vi "Draw Shapes.vi"(0 "Picture in":refnum<vi>, 1 "Commands":cluster{"Time (s)":dbl, T2, "Enabled":bool}[](array[cluster]), 3 "Sample Period (s)":dbl=0.02, 5 "Points":cluster{"x":dbl, "y":dbl, "th":dbl}[](array[cluster]), 6 "Path Points MEGA":cluster{"x":dbl, "y":dbl}[][](array[cluster]), 9 "new picture in":picture, 10 "Output Point MEGA":T1(array[cluster]), 11 "Results":T5, 12 "Output Point":T4, 14 "Path Points":cluster{"x":dbl, "y":dbl}[](array[cluster]), 15 "MEGA?":bool) -> (4 "new picture out":picture)   [LabVIEW 2025]
uses:
  Types/Single Cmd Info.ctl
  <vilib>/picture/picture.llb/imagedata.ctl
  Global Settings.vi
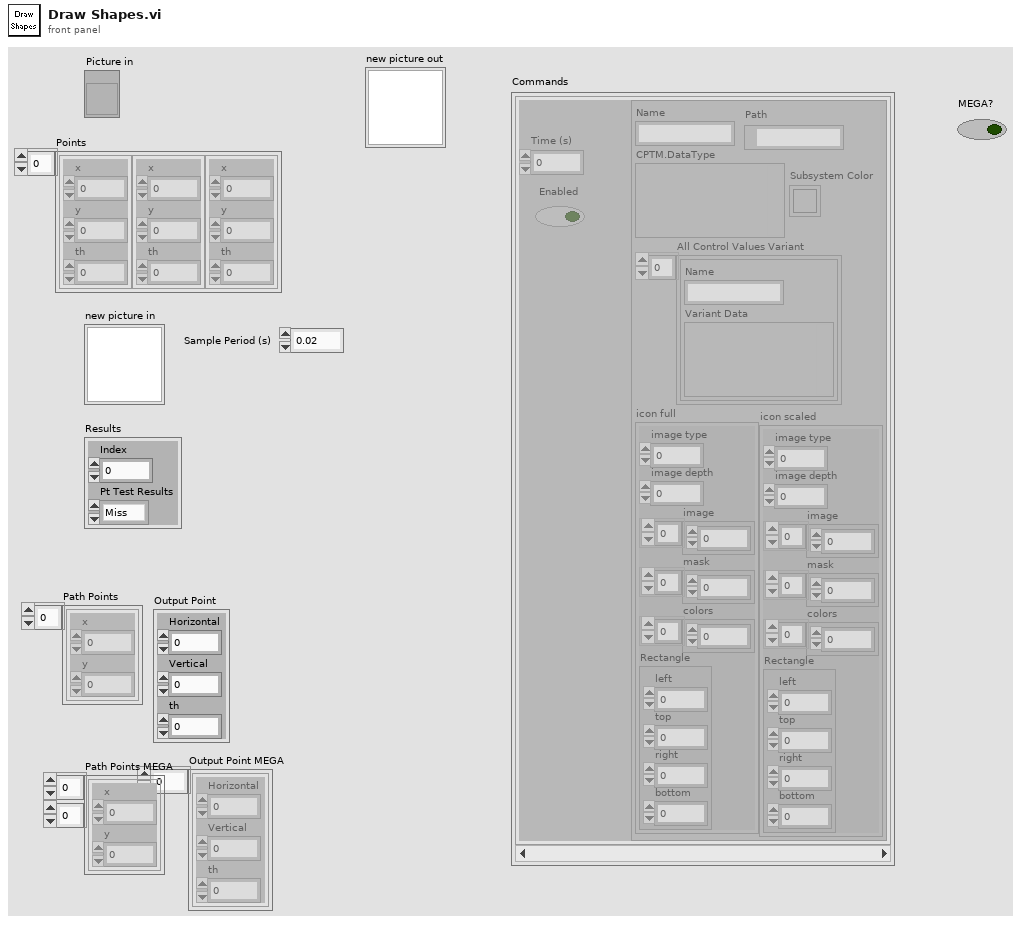
[diagram p1: front panel]
types:
  T1 = cluster{"Horizontal":dbl, "Vertical":dbl, "th":dbl}[]
  T2 = typedef "Single Cmd Info.ctl" = cluster{"Name":string, "CPTM.DataType":variant, "All Control Values Variant":cluster{"Name":string, "Variant Data":variant}[], "icon full":T3, "icon scaled":T3, "Path":path, "Subsystem Color":u32}
  T3 = typedef "imagedata.ctl" = cluster{"image type":i32, "image depth":i32, "image":u8[], "mask":u8[], "colors":u32[], "Rectangle":cluster{"left":i16, "top":i16, "right":i16, "bottom":i16}}
  T4 = cluster{"Horizontal":dbl, "Vertical":dbl, "th":dbl}
  T5 = cluster{"Index":i32, "Pt Test Results":enum16{"Miss", "Rect Hit", "Arrow Hit"}}
  T6 = typedef "LVPositionTypeDef.ctl" = cluster{"Left":i32, "Top":i32}
  T7 = typedef "LVBoundsTypeDef.ctl" = cluster{"Width":u32, "Height":u32}
  T8 = cluster{"left":i16, "top":i16, "right":i16, "bottom":i16}
  T9 = cluster{"Horizontal":dbl, "Vertical":dbl, "Horizontal":dbl, "Vertical":dbl}
  T10 = cluster{i32, "Pt Test Results":enum16{"Miss", "Rect Hit", "Arrow Hit"}}
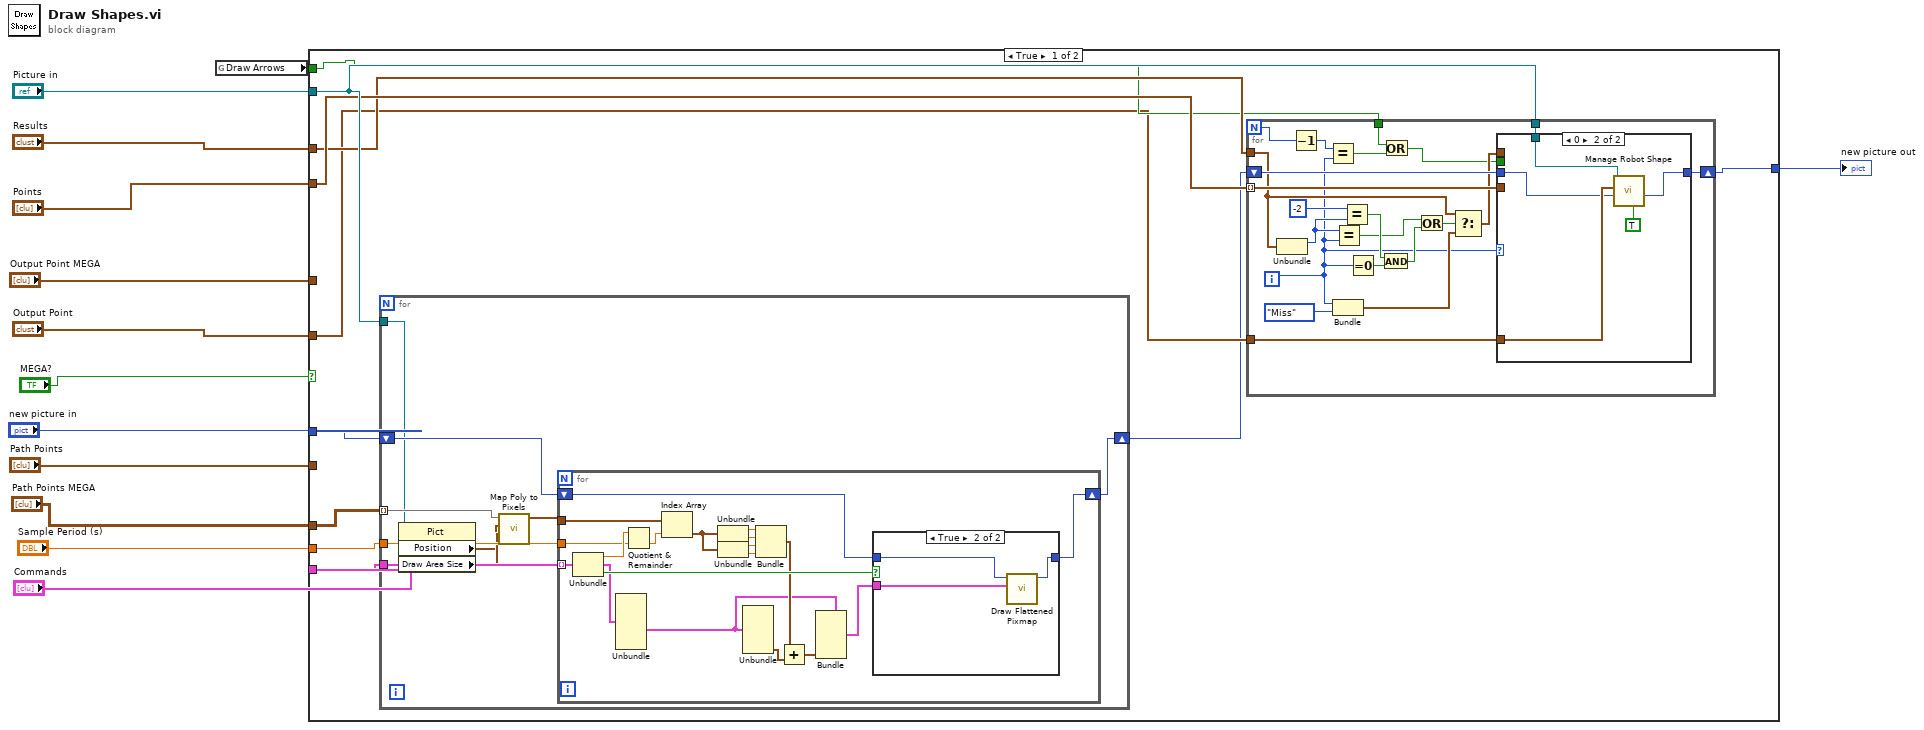
[diagram p0: block diagram]
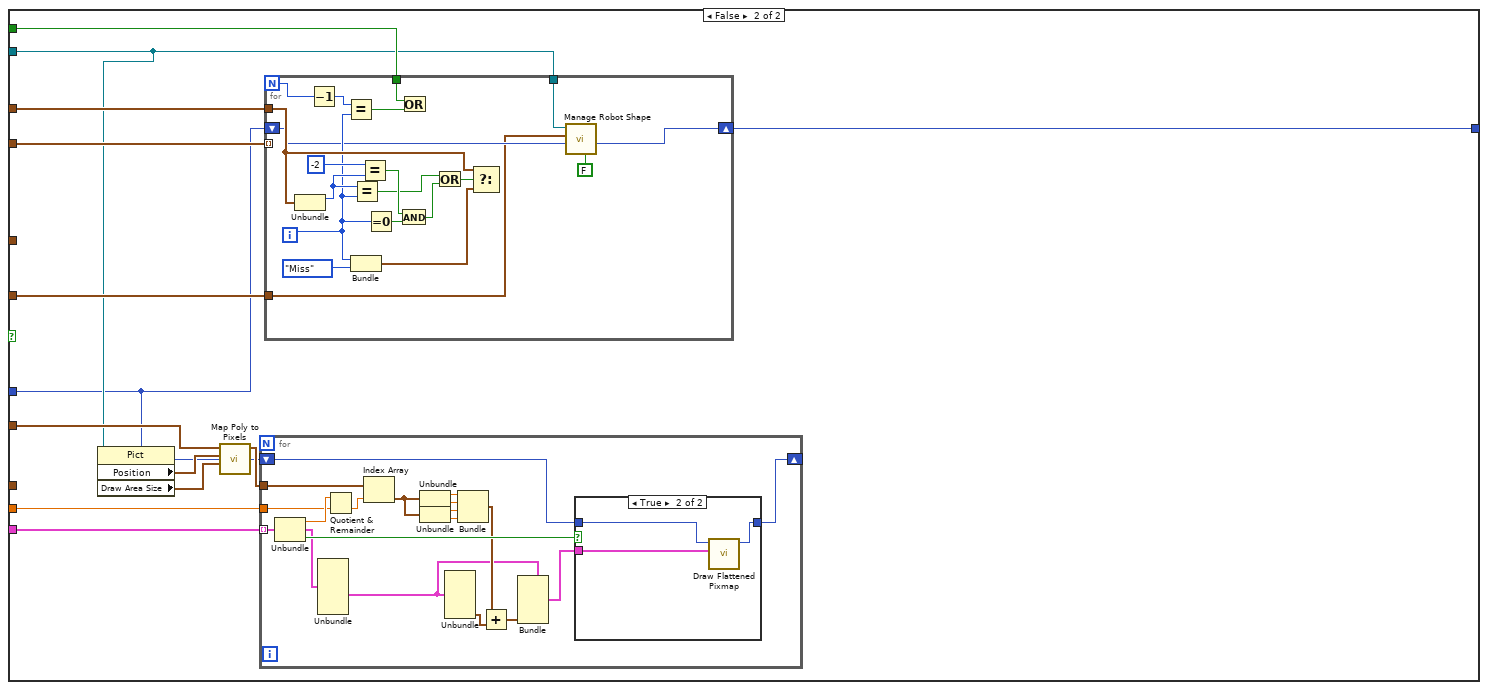
[diagram p4: hidden frame]
diagram:
  n1 = global read "Global Settings.vi" "Draw Arrows"() -> (w5:bool)
  n2 = case shown="True" "MEGA?" {
    tunnel: "Points" -> [w19 w97]
    tunnel: "Results" -> [w18 w96]
    tunnel: "Output Point" -> [w15 w95]
    tunnel: "Sample Period (s)" -> [w24 w94]
    tunnel: "Picture in" -> [w23 w87]
    tunnel: "Commands" -> [w22 w93]
    tunnel: "new picture in" -> [w21 w85]
    tunnel: [w16 w92] -> w6
    tunnel: w5 -> [w17 w91]
    tunnel: "Path Points" -> [_ w88]
    tunnel: "Path Points MEGA" -> [w20 _]
    tunnel: "Output Point MEGA" -> [_ _]
    frame True {
      n3 = for {
        tunnel: w24 -> [w61]
        tunnel: w23 -> [w54]
        tunnel: w20 -> [w55] mode=indexing
        tunnel: w22 -> [w60]
        shift-right: [w53] -> w14
        shift-left: w21 -> [w59]
        n4 = property on="Property Node" class="Pict"(reference=w54) -> ("Position"=w57:T6, "Draw Area Size"=w58:T7)  [unwired: 1 in, 2 out]
        n5 = call "Map Poly to Pixels.vi"("Draw Area Size"=w58, "Position"=w57, "Coords"=w55) -> ("Coords"=w56:cluster{"Horizontal":dbl, "Vertical":dbl}[])  [unwired: 8 in]
        n6 = for {
          shift-right: [w73] -> w53
          shift-left: w59 -> [w75]
          tunnel: w60 -> [w80] mode=indexing
          tunnel: w56 -> [w79]
          tunnel: w61 -> [w77]
          n7 = Unbundle(w80) -> ("Time (s)"=w78:dbl, w71:T2, "Enabled"=w74:bool)
          n8 = Unbundle(w71) -> ("icon scaled"=w63:T3)  [unwired: 6 out]
          n9 = Quotient & Remainder(x=w78, y=w77) -> (floor(x/y)=w76:dbl)  [unwired: 1 out]
          n10 = Index Array(array=w79, index=w76) -> (element=w62:cluster{"Horizontal":dbl, "Vertical":dbl})
          n11 = Unbundle(w62) -> ("Horizontal"=w70:dbl, "Vertical"=w69:dbl)
          n12 = Unbundle(w62) -> ("Horizontal"=w68:dbl, "Vertical"=w67:dbl)
          n13 = Unbundle(w63) -> ("Rectangle"=w65:T8)  [unwired: 5 out]
          n14 = Bundle("Horizontal"=w70, "Vertical"=w69, "Horizontal"=w68, "Vertical"=w67) -> (w64:T9)  [unwired: 1 in]
          n15 = Add(x=w64, y=w65) -> (x+y=w72:cluster{dbl, dbl, dbl, dbl})
          n16 = Bundle(cluster=w63, "Rectangle"=w72) -> (w66:T3)  [unwired: 5 in]
          n17 = case shown="True" w74 {
            tunnel: [w81 w82] -> w73
            tunnel: w75 -> [w81 w83]
            tunnel: w66 -> [_ w84]
            frame False {
            }
            frame True {
              n18 = call <vilib>:"Draw Flattened Pixmap.vi"("image data"=w84, "picture"=w83) -> ("new picture"=w82:picture)  [unwired: 7 in]
            }
          }
        }
      }
      n19 = for {
        N -> [w31]
        tunnel: w19 -> [w46] mode=indexing
        shift-right: [w45] -> w16
        shift-left: w14 -> [w44]
        tunnel: w23 -> [w43]
        tunnel: w18 -> [w40]
        tunnel: w15 -> [w28]
        tunnel: w17 -> [w25]
        i -> [w29]
        n20 = Unbundle(w40) -> ("Index"=w36:i32)  [unwired: 1 out]
        n21 = Decrement(x=w31) -> (x-1=w30:i32)
        n22 = Equal?(x=w30, y=w29) -> (x = y?=w27:bool)
        n23 = Bundle(w29, "Pt Test Results"=enum16{"Miss", "Rect Hit", "Arrow Hit"}."Miss") -> (w41:T10)  [unwired: 1 in]
        n24 = Equal?(x=w36, y=w29) -> (x = y?=w33:bool)
        n25 = Equal?(x=-2, y=w36) -> (x = y?=w35:bool)
        n26 = Equal To 0?(x=w29) -> (x = 0?=w38:bool)
        n27 = And(x=w35, y=w38) -> (x .and. y?=w34:bool)
        n28 = Or(x=w25, y=w27) -> (x .or. y?=w26:bool)
        n29 = Or(x=w33, y=w34) -> (x .or. y?=w32:bool)
        n30 = Select(t=w40, s=w32, f=w41) -> (s? t:f=w42:T5)
        n31 = case shown="0" w29 {
          tunnel: w46 -> [_ _]
          tunnel: [w47 w52] -> w45
          tunnel: w44 -> [w47 w48]
          tunnel: w43 -> [_ w50]
          tunnel: w42 -> [_ _]
          tunnel: w26 -> [_ _]
          tunnel: w28 -> [_ w51]
          frame Default {
          }
          frame 0 {
            n32 = call "Manage Robot Shape.vi"("Lighter"=TRUE ("Outline"), "new picture in"=w48, "Robot Position (ft)"=w51, "Pict Ref"=w50) -> ("new picture out"=w52:picture)  [unwired: 5 in, 2 out]
          }
        }
      }
    }
    frame False {
      n33 = property on="Property Node" class="Pict"(reference=w87) -> ("Position"=w90:T6, "Draw Area Size"=w89:T7)  [unwired: 1 in, 2 out]
      n34 = call "Map Poly to Pixels.vi"("Draw Area Size"=w89, "Position"=w90, "Coords"=w88) -> ("Coords"=w86:cluster{"Horizontal":dbl, "Vertical":dbl}[])  [unwired: 8 in]
      n35 = for {
        shift-right: [w109] -> _
        shift-left: w85 -> [w111]
        tunnel: w93 -> [w116] mode=indexing
        tunnel: w86 -> [w115]
        tunnel: w94 -> [w113]
        n36 = Unbundle(w116) -> ("Time (s)"=w114:dbl, w107:T2, "Enabled"=w110:bool)
        n37 = Unbundle(w107) -> ("icon scaled"=w99:T3)  [unwired: 6 out]
        n38 = Quotient & Remainder(x=w114, y=w113) -> (floor(x/y)=w112:dbl)  [unwired: 1 out]
        n39 = Index Array(array=w115, index=w112) -> (element=w98:cluster{"Horizontal":dbl, "Vertical":dbl})
        n40 = Unbundle(w98) -> ("Horizontal"=w106:dbl, "Vertical"=w105:dbl)
        n41 = Unbundle(w98) -> ("Horizontal"=w104:dbl, "Vertical"=w103:dbl)
        n42 = Unbundle(w99) -> ("Rectangle"=w101:T8)  [unwired: 5 out]
        n43 = Bundle("Horizontal"=w106, "Vertical"=w105, "Horizontal"=w104, "Vertical"=w103) -> (w100:T9)  [unwired: 1 in]
        n44 = Add(x=w100, y=w101) -> (x+y=w108:cluster{dbl, dbl, dbl, dbl})
        n45 = Bundle(cluster=w99, "Rectangle"=w108) -> (w102:T3)  [unwired: 5 in]
        n46 = case shown="True" w110 {
          tunnel: [w117 w118] -> w109
          tunnel: w111 -> [w117 w119]
          tunnel: w102 -> [_ w120]
          frame False {
          }
          frame True {
            n47 = call <vilib>:"Draw Flattened Pixmap.vi"("image data"=w120, "picture"=w119) -> ("new picture"=w118:picture)  [unwired: 7 in]
          }
        }
      }
      n48 = for {
        N -> [w130]
        tunnel: w97 -> [_] mode=indexing
        shift-right: [w123] -> w92
        shift-left: w85 -> [w125]
        tunnel: w87 -> [w124]
        tunnel: w96 -> [w139]
        tunnel: w95 -> [w122]
        tunnel: w91 -> [w126]
        i -> [w128]
        n49 = Unbundle(w139) -> ("Index"=w135:i32)  [unwired: 1 out]
        n50 = Decrement(x=w130) -> (x-1=w129:i32)
        n51 = Equal?(x=w129, y=w128) -> (x = y?=w127:bool)
        n52 = Bundle(w128, "Pt Test Results"=enum16{"Miss", "Rect Hit", "Arrow Hit"}."Miss") -> (w140:T10)  [unwired: 1 in]
        n53 = Equal?(x=w135, y=w128) -> (x = y?=w132:bool)
        n54 = Equal?(x=-2, y=w135) -> (x = y?=w134:bool)
        n55 = Equal To 0?(x=w128) -> (x = 0?=w137:bool)
        n56 = And(x=w134, y=w137) -> (x .and. y?=w133:bool)
        n57 = Or(x=w126, y=w127) -> ()  [unwired: 1 out]
        n58 = Or(x=w132, y=w133) -> (x .or. y?=w131:bool)
        n59 = Select(t=w139, s=w131, f=w140) -> ()  [unwired: 1 out]
        n60 = call "Manage Robot Shape.vi"("Lighter"=FALSE, "new picture in"=w125, "Robot Position (ft)"=w122, "Pict Ref"=w124) -> ("new picture out"=w123:picture)  [unwired: 5 in, 2 out]
      }
    }
  }
  "new picture out" <- w6
